vi "Test Controller Depositing after Calling Deposit.vi"(8 "error in (no error)":errorcluster, 11 "Test Case In":refnum<class "Controller Test.lvclass">) -> (0 "error out":errorcluster, 3 "Test Case Out":refnum<class "Controller Test.lvclass">)   [LabVIEW 2020, in "Controller Test.lvclass"]
uses:
  Controller Test.lvclass
  Controller Test.lvclass/Controller Test.ctl
  01074fa8-ee8a-411d-bc8b-fc92c4f90959.vi
  ATM Controller/ATM Controller.lvclass
  ATM Controller/State.ctl
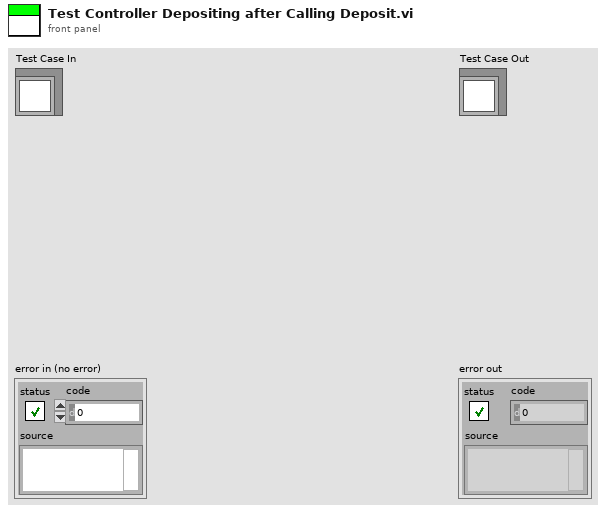
[diagram p1: front panel]
types:
  T1 = typedef "ATM Controller.lvclass/State.ctl" = enum16{"Start", "Card Inserted", "Verification Failed", "Verification Succeeded", "Depositing", "Terminate"}
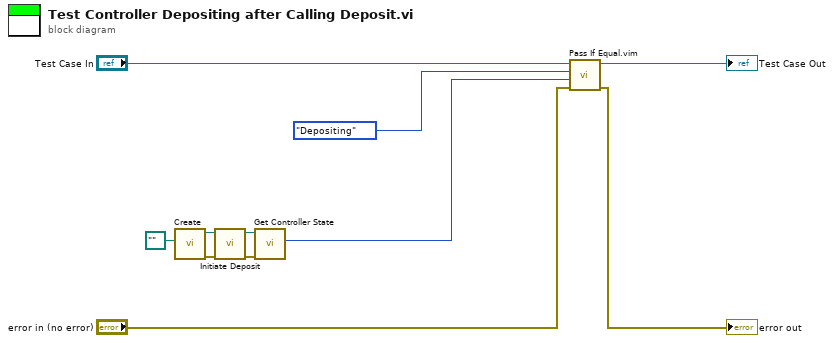
[diagram p0: block diagram]
diagram:
  n1 = call "Create.vi"("Data File"=path "") -> ("error out"=w7:errorcluster, "ATM Controller out"=w2:refnum<class "ATM Controller.lvclass">)  [unwired: 9 in]
  n2 = call "Initiate Deposit.vi"("error in (no error)"=w7, "ATM Controller in"=w2) -> ("error out"=w3:errorcluster, "ATM Controller out"=w1:refnum<class "ATM Controller.lvclass">)  [unwired: 8 in]
  n3 = call "Get Controller State.vi"("error in (no error)"=w3, "ATM Controller in"=w1) -> ("ATM State"=w6:T1)  [unwired: 7 in, 2 out]
  n4 = call "Pass If Equal.vim"("error in (no error)"="error in (no error)", "Actual"=w6, "Expected"=State."Depositing" ("ATM State"), "LUnit Test Case In"="Test Case In") -> ("error out"=→"error out":errorcluster, "LUnit Test Case Out"=→"Test Case Out":refnum<class "Controller Test.lvclass">)  [unwired: 6 in]
